vi "Password_RePrompt.vi"(8 "Status/Errors in":refnum<vi>, 9 "Wrong password?":bool) -> (0 "Status/Errors out":refnum<vi>, 1 "OK button?":bool, 2 "Password":string)   [LabVIEW 2013]
uses:
  Instance           2 25Saved   Password_RePrompt .vi
  Instance           1 25Saved   Password_RePrompt .vi
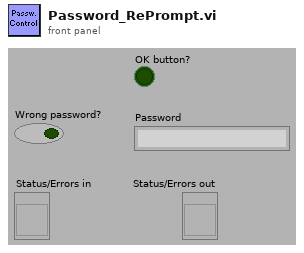
[diagram p1: front panel]
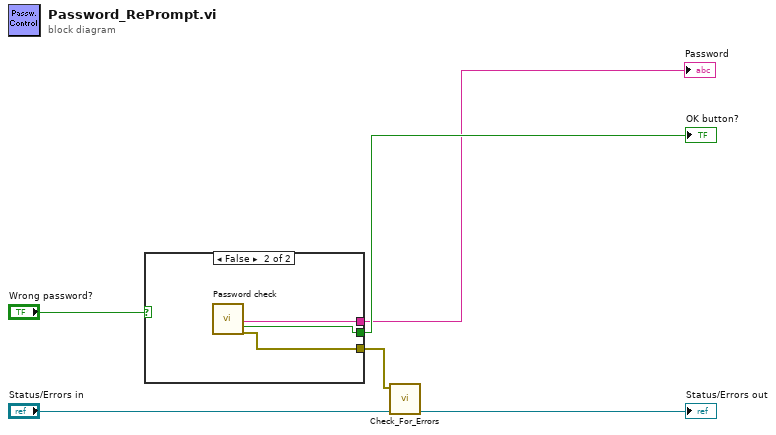
[diagram p0: block diagram]
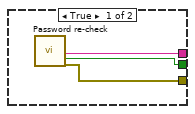
[diagram p2: hidden frame]
diagram:
  n1 = case shown="False" "Wrong password?" {
    tunnel: [w9 w12] -> w1
    tunnel: [w7 w11] -> w3
    tunnel: [w8 w10] -> w2
    frame True {
      n2 = call "Password re-check"() -> ("Password"=w9:string, "OK"=w8:bool, "error out"=w7:errorcluster)  [unwired: 3 in, 14 out]
    }
    frame False {
      n3 = call "Password check"() -> ("Password"=w12:string, "OK"=w10:bool, "error out"=w11:errorcluster)  [unwired: 3 in, 14 out]
    }
  }
  "OK button?" <- w2
  "Password" <- w1
  n4 = call "Check_For_Errors.vi"("Status/Errors in"="Status/Errors in", "error in"=w3) -> ("Status/Errors out"=→"Status/Errors out":refnum<vi>)  [unwired: 9 out]
